vi "test5160ExtraSamples.vi"() -> ()   [LabVIEW 2013]
panel:
  out "Waveform Graph 3":dbl[](graph)
  out "Waveform Graph":dbl[](graph)
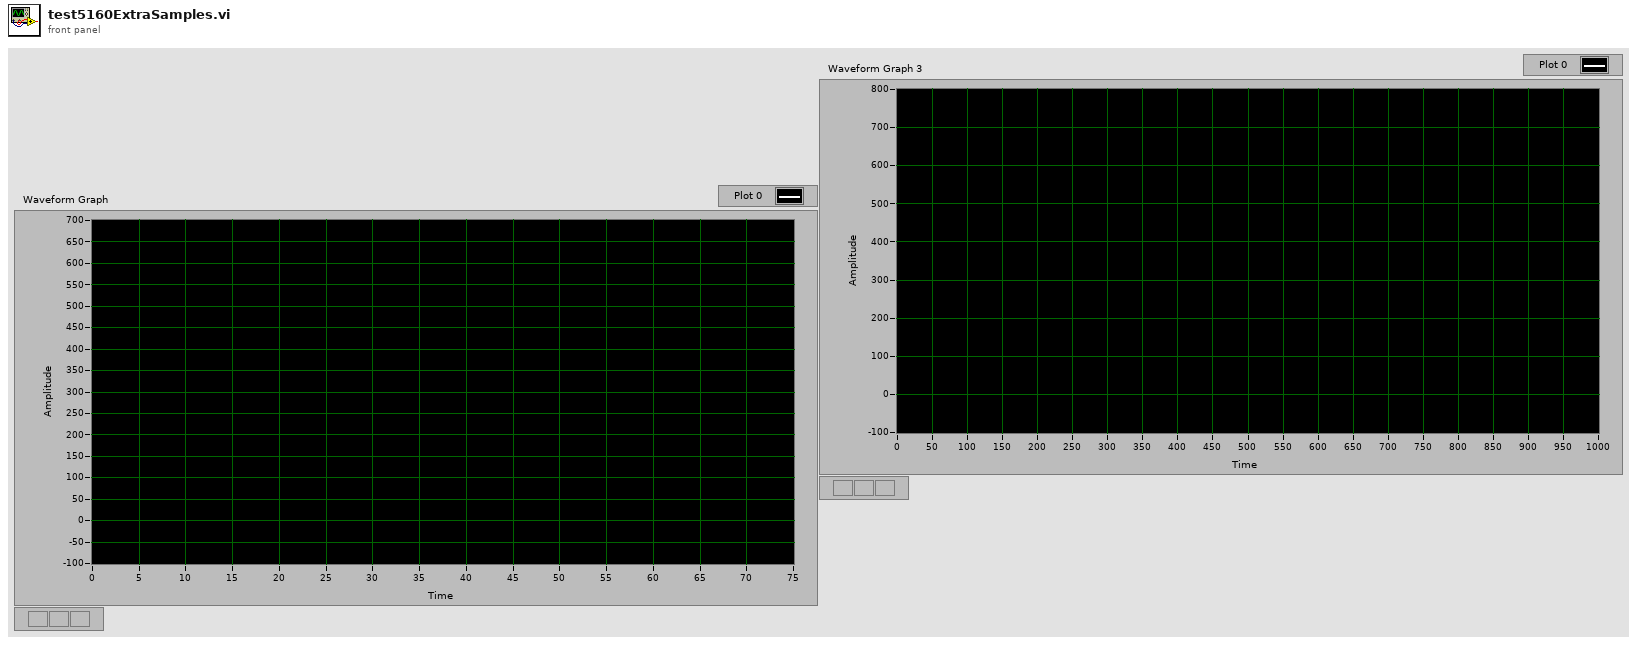
[diagram p1: front panel]
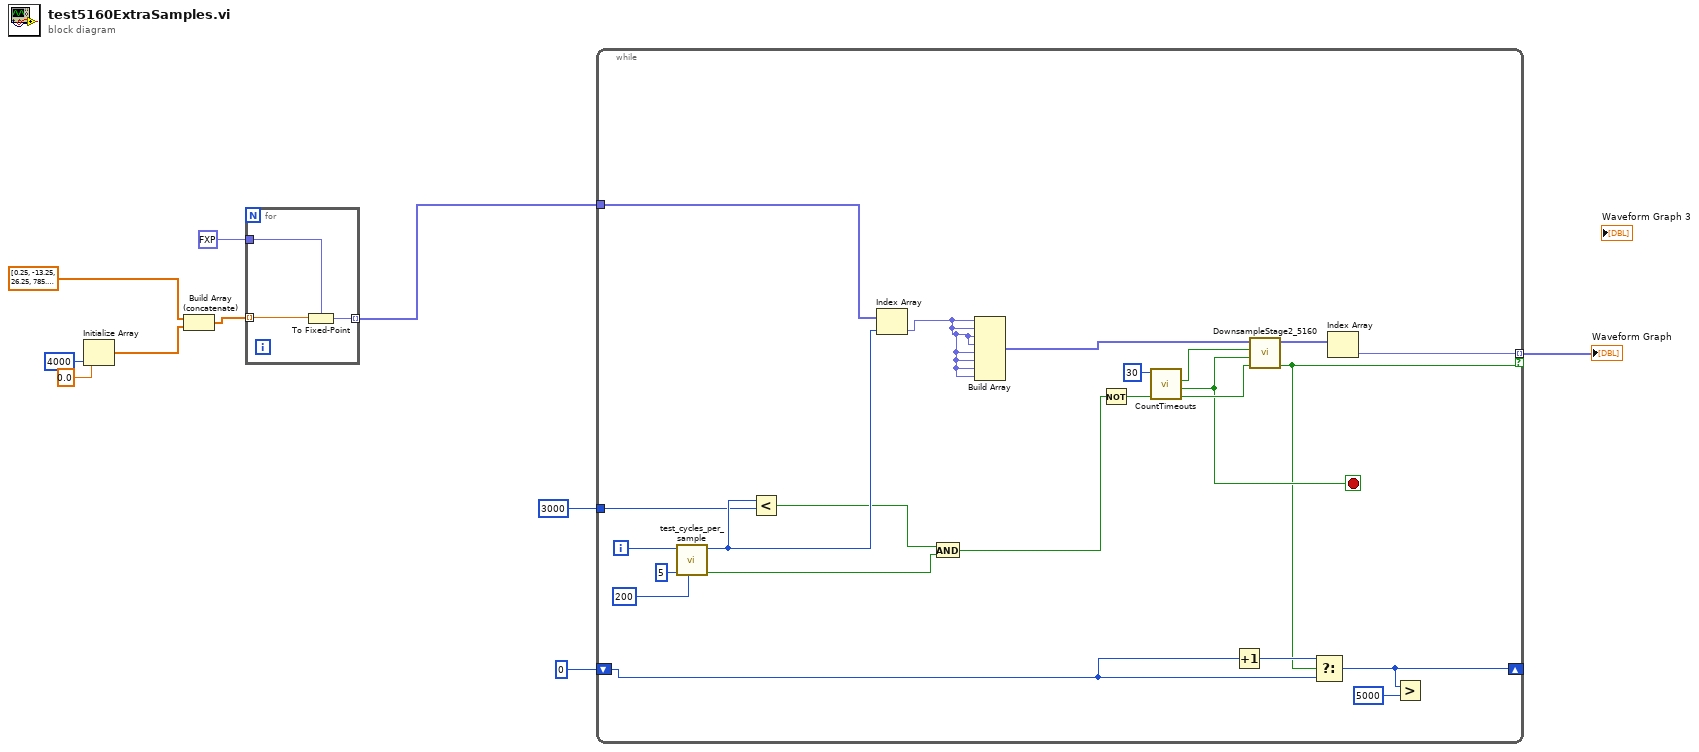
[diagram p0: block diagram]
diagram:
  n1 = Initialize Array(0.0 ("element"), 4000 ("dimension size")) -> (w8:dbl[])
  n2 = Build Array (concatenate)(dbl[] [0.25, -13.25, 26.25, 785.5, 502.0, 744.75, 566.25, 612.25, 716.25, 502.0, 744.75, 566.25, 612.25, 716.25, 502.0, 744.75, 566.25, 612.25, 716.25, 502.0, 744.75, 566.25, 612.25, 716.25, 502.0, 744.75, 566.25, 612.25, 716.25, 502.0, 744.75, 566.25, 612.25, 716.25, 502.0, 744.75, 566.25, 612.25, 716.25, 502.0, 744.75, 566.25, 612.25, 716.25, 502.0, 744.75, 566.25, 612.25, 716.25, 502.0, 744.75, 566.25, 612.25, 716.25, 502.0, 744.75, 566.25, 612.25, 716.25, 502.0, 744.75, 566.25, 612.25, 716.25, 502.0, 744.75, 566.25, 612.25, 716.25, 502.0, 744.75, 566.25, 612.25, 716.25, 502.0, 744.75, 566.25, 612.25, 716.25, 502.0, 744.75, 566.25, 612.25, 716.25, 502.0, 744.75, 566.25, 612.25, 716.25, 502.0, 744.75, 566.25, 612.25, 716.25, 502.0, 744.75, 566.25, 612.25, 716.25, 502.0, 744.75, 566.25, 612.25, 716.25, 502.0, 744.75, 566.25, 612.25, 716.25, 502.0, 744.75, 566.25, 612.25, 716.25, 502.0, 744.75, 566.25, 612.25, 716.25, 502.0, 744.75, 566.25, 612.25, 716.25, 502.0, 744.75, 566.25, 612.25, 716.25, 502.0, 744.75, 566.25, 612.25, 716.25, 502.0, 744.75, 566.25, 612.25, 716.25, 502.0, 744.75, 566.25, 612.25, 716.25, 502.0, 744.75, 566.25, 612.25, 716.25, 502.0, 744.75, 566.25, 612.25, 716.25, 502.0, 744.75, 566.25, 612.25, 716.25, 502.0, 744.75, 566.25, 612.25, 716.25, 502.0, 744.75, 566.25, 612.25, 716.25, 502.0, 744.75, 566.25, 612.25, 716.25, 502.0, 744.75, 566.25, 612.25, 716.25, 502.0, 744.75, 566.25, 612.25, 716.25, 502.0, 744.75, 566.25, 612.25, 716.25, 502.0, 744.75, 566.25, 612.25, 716.25, 502.0, 744.75, 566.25, 612.25, 716.25, 502.0, 744.75, 566.25, 612.25, 716.25, 502.0, 744.75, 566.25, 612.25, 716.25, 502.0, 744.75, 566.25, 612.25, 716.25, 502.0, 744.75, 566.25, 612.25, 716.25, 502.0, 744.75, 566.25, 612.25, 716.25, 502.0, 744.75, 566.25, 612.25, 716.25, 502.0, 744.75, 566.25, 612.25, 716.25, 502.0, 744.75, 566.25, 612.25, 716.25, 502.0, 744.75, 566.25, 612.25, 716.25, 502.0, 744.75, 566.25, 612.25, 716.25, 502.0, 744.75, 566.25, 612.25, 716.25, 502.0, 744.75, 566.25, 612.25, 716.25, 502.0, 744.75, 566.25, 612.25, 716.25, 502.0, 744.75, 566.25, 612.25, 716.25, 502.0, 744.75, 566.25, 612.25, 716.25, 502.0, 744.75, 566.25, 612.25, 716.25, 502.0, 744.75, 566.25, 612.25, 716.25, 502.0, 744.75, 566.25, 612.25, 716.25, 502.0, 744.75, 566.25, 612.25, 716.25, 502.0, 744.75, 566.25, 612.25, 716.25, 502.0, 744.75, 566.25, 612.25, 716.25, 502.0, 744.75, 566.25, 612.25, 716.25, 502.0, 744.75, 566.25, 612.25, 716.25, 502.0, 744.75, 566.25, 612.25, 716.25, 502.0, 744.75, 566.25, 612.25, 716.25, 502.0, 744.75, 566.25, 612.25, 716.25, 502.0, 744.75, 566.25, 612.25, 716.25, 502.0, 744.75, 566.25, 612.25, 716.25, 502.0, 744.75, 566.25, 612.25, 716.25, 502.0, 744.75, 566.25, 612.25, 716.25, 502.0, 744.75, 566.25, 612.25, 716.25, 502.0, 744.75, 566.25, 612.25, 716.25, 502.0, 744.75, 566.25, 612.25, 716.25, 502.0, 744.75, 566.25, 612.25, 716.25, 502.0, 744.75, 566.25, 612.25, 716.25, 502.0, 744.75, 566.25, 612.25, 716.25, 502.0, 744.75, 566.25, 612.25, 716.25, 502.0, 744.75, 566.25, 612.25, 716.25, 502.0, 744.75, 566.25, 612.25, 716.25, 502.0, 744.75, 566.25, 612.25, 716.25, 502.0, 744.75, 566.25, 612.25, 716.25, 502.0, 744.75, 566.25, 612.25, 716.25, 502.0, 744.75, 566.25, 612.25, 716.25, 502.0, 744.75, 566.25, 612.25, 716.25, 502.0, 744.75, 566.25, 612.25, 716.25, 502.0, 744.75, 566.25, 612.25, 716.25, 502.0, 744.75, 566.25, 612.25, 716.25, 502.0, 744.75, 566.25, 612.25, 716.25, 502.0, 744.75, 566.25, 612.25, 716.25, 502.0, 744.75, 566.25, 612.25, 716.25, 502.0, 744.75, 566.25, 612.25, 716.25, 502.0, 744.75, 566.25, 612.25, 716.25, 502.0, 744.75, 566.25, 612.25, 716.25, 502.0, 744.75, 566.25, 612.25, 716.25, 502.0, 744.75, 566.25, 612.25, 716.25, 502.0, 744.75, 566.25, 612.25, 716.25, 502.0, 744.75, 566.25, 612.25, 716.25, 502.0, 744.75, 566.25, 612.25, 716.25, 502.0, 744.75, 566.25, 612.25, 716.25, 502.0, 744.75, 566.25, 612.25, 716.25, 502.0, 744.75, 566.25, 612.25, 716.25, 502.0, 744.75, 566.25, 612.25, 716.25, 502.0, 744.75, 566.25, 612.25, 716.25, 502.0, 744.75, 566.25, 612.25, 716.25, 502.0, 744.75, 566.25, 612.25, 716.25, 502.0, 744.75, 566.25, 612.25, 716.25, 502.0, 744.75, 566.25, 612.25, 716.25, 502.0, 744.75, 566.25, 612.25, 716.25, 502.0, 744.75, 566.25, 612.25, 716.25, 502.0, 744.75, 566.25, 612.25, 716.25, 502.0, 744.75, 566.25, 612.25, 716.25, 502.0, 744.75, 566.25, 612.25, 716.25, 502.0, 744.75, 566.25, 612.25, 716.25, 502.0, 744.75, 566.25, 612.25, 716.25, 502.0, 744.75, 566.25, 612.25, 716.25, 502.0, 744.75, 566.25, 612.25, 716.25, 502.0, 744.75, 566.25, 612.25, 716.25, 502.0, 744.75, 566.25, 612.25, 716.25, 502.0, 744.75, 566.25, 612.25, 716.25, 502.0, 744.75, 566.25, 612.25, 716.25, 502.0, 744.75, 566.25, 612.25, 716.25, 502.0, 744.75, 566.25, 612.25, 716.25, 502.0, 744.75, 566.25, 612.25, 716.25, 502.0, 744.75, 566.25, 612.25, 716.25, 502.0, 744.75, 566.25, 612.25, 716.25, 502.0, 744.75, 566.25, 612.25, 716.25, 502.0, 744.75, 566.25, 612.25, 716.25, 502.0, 744.75, 566.25, 612.25, 716.25, 502.0, 744.75, 566.25, 612.25, 716.25, 502.0, 744.75, 566.25, 612.25, 716.25, 502.0, 744.75, 566.25, 612.25, 716.25, 502.0, 744.75, 566.25, 612.25, 716.25, 502.0, 744.75, 566.25, 612.25, 716.25, 502.0, 744.75, 566.25, 612.25, 716.25, 502.0, 744.75, 566.25, 612.25, 716.25, 502.0, 744.75, 566.25, 612.25, 716.25, 502.0, 744.75, 566.25, 612.25, 716.25, 502.0, 744.75, 566.25, 612.25, 716.25, 502.0, 744.75, 566.25, 612.25, 716.25, 502.0, 744.75, 566.25, 612.25, 716.25, 502.0, 744.75, 566.25, 612.25, 716.25, 502.0, 744.75, 566.25, 612.25, 716.25, 502.0, 744.75, 566.25, 612.25, 716.25, 502.0, 744.75, 566.25, 612.25, 716.25, 502.0, 744.75, 566.25, 612.25, 716.25, 502.0, 744.75, 566.25, 612.25, 716.25, 502.0, 744.75, 566.25, 612.25, 716.25, 502.0, 744.75, 566.25, 612.25, 716.25, 502.0, 744.75, 566.25, 612.25, 716.25, 502.0, 744.75, 566.25, 612.25, 716.25, 502.0, 744.75, 566.25, 612.25, 716.25, 502.0, 744.75, 566.25, 612.25, 716.25, 502.0, 744.75, 566.25, 612.25, 716.25, 502.0, 744.75, 566.25, 612.25, 716.25, 502.0, 744.75, 566.25, 612.25, 716.25, 502.0, 744.75, 566.25, 612.25, 716.25, 502.0, 744.75, 566.25, 612.25, 716.25, 502.0, 744.75, 566.25, 612.25, 716.25, 502.0, 744.75, 566.25, 612.25, 716.25, 502.0, 744.75, 566.25, 612.25, 716.25, 502.0, 744.75, 566.25, 612.25, 716.25, 502.0, 744.75, 566.25, 612.25, 716.25, 502.0, 744.75, 566.25, 612.25, 716.25, 502.0, 744.75, 566.25, 612.25, 716.25, 502.0, 744.75, 566.25, 612.25, 716.25, 502.0, 744.75, 566.25, 612.25, 716.25, 502.0, 744.75, 566.25, 612.25, 716.25, 502.0, 744.75, 566.25, 612.25, 716.25, 502.0, 744.75, 566.25, 612.25, 716.25, 502.0, 744.75, 566.25, 612.25, 716.25, 502.0, 744.75, 566.25, 612.25, 716.25, 502.0, 744.75, 566.25, 612.25, 716.25, 502.0, 744.75, 566.25, 612.25, 716.25, 502.0, 744.75, 566.25, 612.25, 716.25, 502.0, 744.75, 566.25, 612.25, 716.25, 502.0, 744.75, 566.25, 612.25, 716.25, 502.0, 744.75, 566.25, 612.25, 716.25, 502.0, 744.75, 566.25, 612.25, 716.25, 502.0, 744.75, 566.25, 612.25, 716.25, 502.0, 744.75, 566.25, 612.25, 716.25, 502.0, 744.75, 566.25, 612.25, 716.25, 502.0, 744.75, 566.25, 612.25, 716.25, 502.0, 744.75, 566.25, 612.25, 716.25, 502.0, 744.75, 566.25, 612.25, 716.25, 502.0, 744.75, 566.25, 612.25, 716.25, 502.0, 744.75, 566.25, 612.25, 716.25, 502.0, 744.75, 566.5, 612.25, 716.25, 502.0, 744.75, 566.5, 612.25, 716.25, 502.0, 744.75, 566.5, 612.25, 716.25, 502.0, 744.75, 566.5, 612.25, 716.25, 502.0, 744.75, 566.5, 612.25, 716.25, 502.0, 744.75, 566.5, 612.25, 716.25, 502.0, 744.75, 579.5, 571.25, -74.75, 0.5, 0.0, 0.0, 0.0, 0.0, 0.0, 0.0, 0.0, 0.0, 0.0, 0.0, 0.0, 0.0, 0.0, 0.0, 0.0, 0.0, 0.0, 0.0, 0.0, 0.0, 0.0, 0.0, 0.0, 0.0, 0.0, 0.0, 0.0, 0.0, 0.0, 0.0, 0.0, 0.0, 0.0, 0.0, 0.0, 0.0] ("Waveform Graph 3"), w8) -> (w4:dbl[])
  n3 = for {
    tunnel: w4 -> [w11] mode=indexing
    tunnel: fxp<+/-,16,14> 0.0 ("Q out") -> [w13]
    tunnel: [w12] -> w3 mode=indexing
    n4 = To Fixed-Point(fixed-point type=w13, number=w11) -> (fixed-point=w12:fxp<+/-,16,14>)
  }
  n5 = while {
    shift-right: [w30] -> _
    shift-left: 0 ("initial delay") -> [w33]
    tunnel: [w31] -> w5 mode=indexing if=w19
    tunnel: w3 -> [w23]
    tunnel: 3000 ("y") -> [w17]
    i -> [w29]
    stop <- w20 stop-if-true
    n6 = call "test_cycles_per_sample.vi"("initial delay"=200, "cycles per sample"=5, "index"=w29) -> ("valid out"=w15:bool, "array index"=w18:i32)  [unwired: 7 in]
    n7 = Less?(x=w18, y=w17) -> (x < y?=w16:bool)
    n8 = Index Array(array=w23, index=w18) -> (element=w22:fxp<+/-,16,14>)
    n9 = And(x=w16, y=w15) -> (x .and. y?=w14:bool)
    n10 = Build Array(w22, w22, w22, w22, w22, w22, w22, w22) -> (w21:fxp<+/-,16,14>[])
    n11 = Not(x=w14) -> (.not. x?=w24:bool)
    n12 = call "CountTimeouts.vi"("Timed out"=w24, "Extra samples"=i16 30) -> ("Valid sample"=w25:bool, "Reset"=w20:bool, "Extra sample"=w26:bool)  [unwired: 7 in]
    n13 = Increment(x=w33) -> (x+1=w34:i32)
    n14 = call "DownsampleStage2_5160.vi"("valid in"=w25, "reset"=w20, "extra sample"=w26, "Element"=w21) -> ("valid out"=w19:bool, "Array"=w28:fxp<+/-,16,14>[])  [unwired: 6 in]
    n15 = Select(t=w34, s=w19, f=w33) -> (s? t:f=w30:i32)
    n16 = Index Array(array=w28) -> (element=w31:fxp<+/-,16,14>)  [unwired: 1 in]
    n17 = Greater?(x=w30, y=5000) -> ()  [unwired: 1 out]
  }
  "Waveform Graph" <- w5
